vi "VIP_Post-Install Custom Action.vi"(10 "Variant":variant) -> (0 "error out":errorcluster)   [LabVIEW 2020]
uses:
  <vilib>/Utility/sysdir.llb/System Directory Type.ctl
  <userlib>/_OpenG.lib/file/file.llb/openg_file.lvlib
  <userlib>/_OpenG.lib/file/file.llb/Build Path - Traditional__ogtk.vi
  <userlib>/_OpenG.lib/lvzip/fileutil.llb/subVIs/FILE Rename (Path)__ogtk.vi
  <userlib>/_OpenG.lib/file/file.llb/File Exists - Scalar__ogtk.vi
panel:
  # "POST INSTALL"
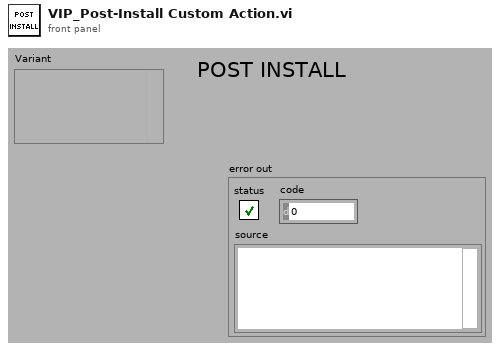
[diagram p1: front panel]
types:
  T1 = enum16{"open", "replace", "create", "open or create", "replace or create", "replace or create with confirmation"}
  T2 = typedef "System Directory Type.ctl" = i32
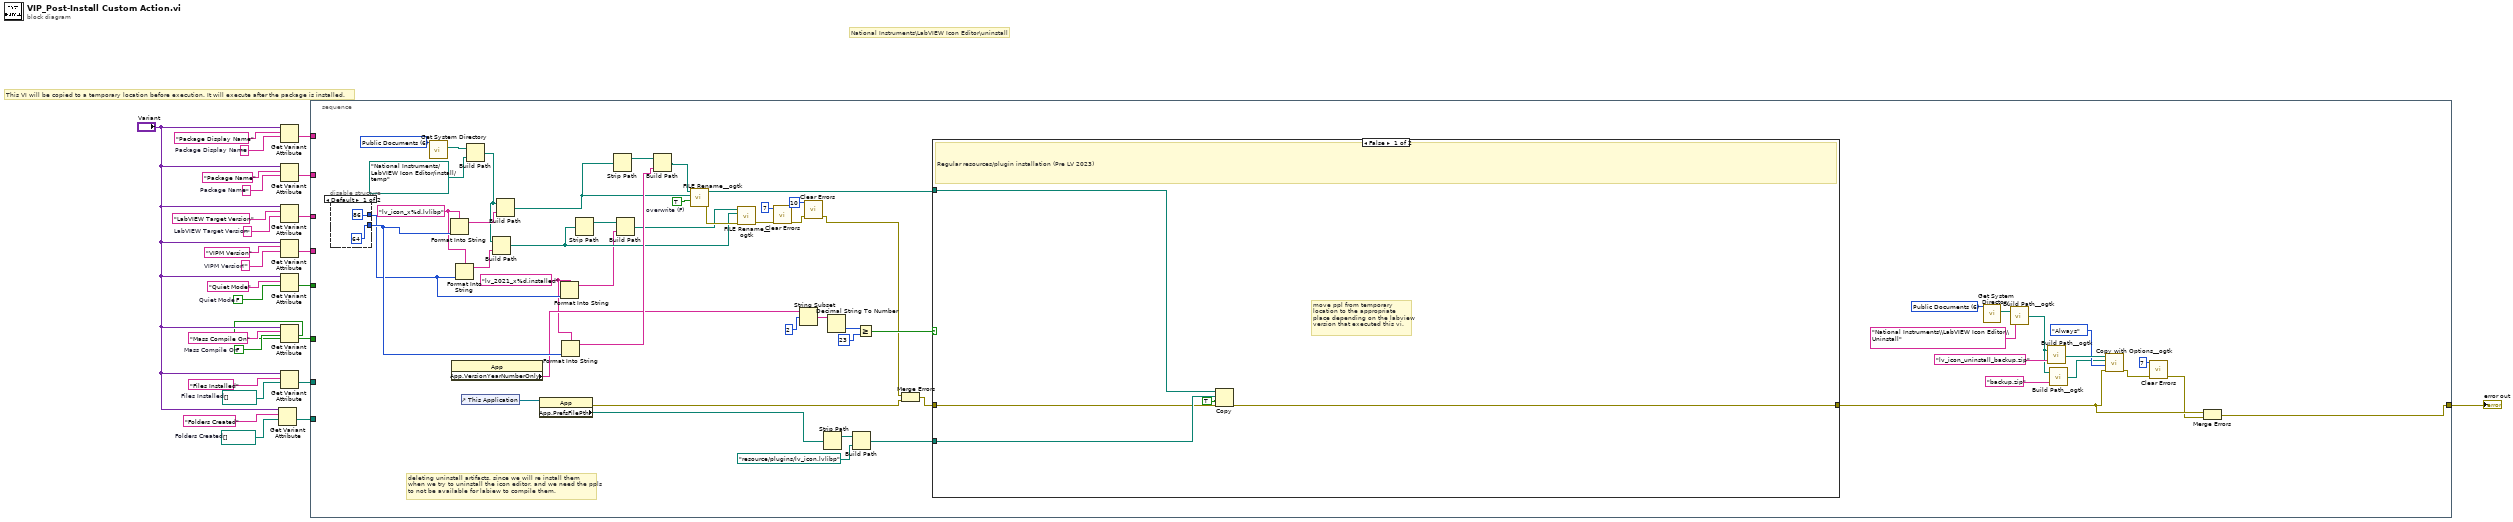
[diagram p0: block diagram]
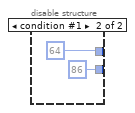
[diagram p2: hidden frame]
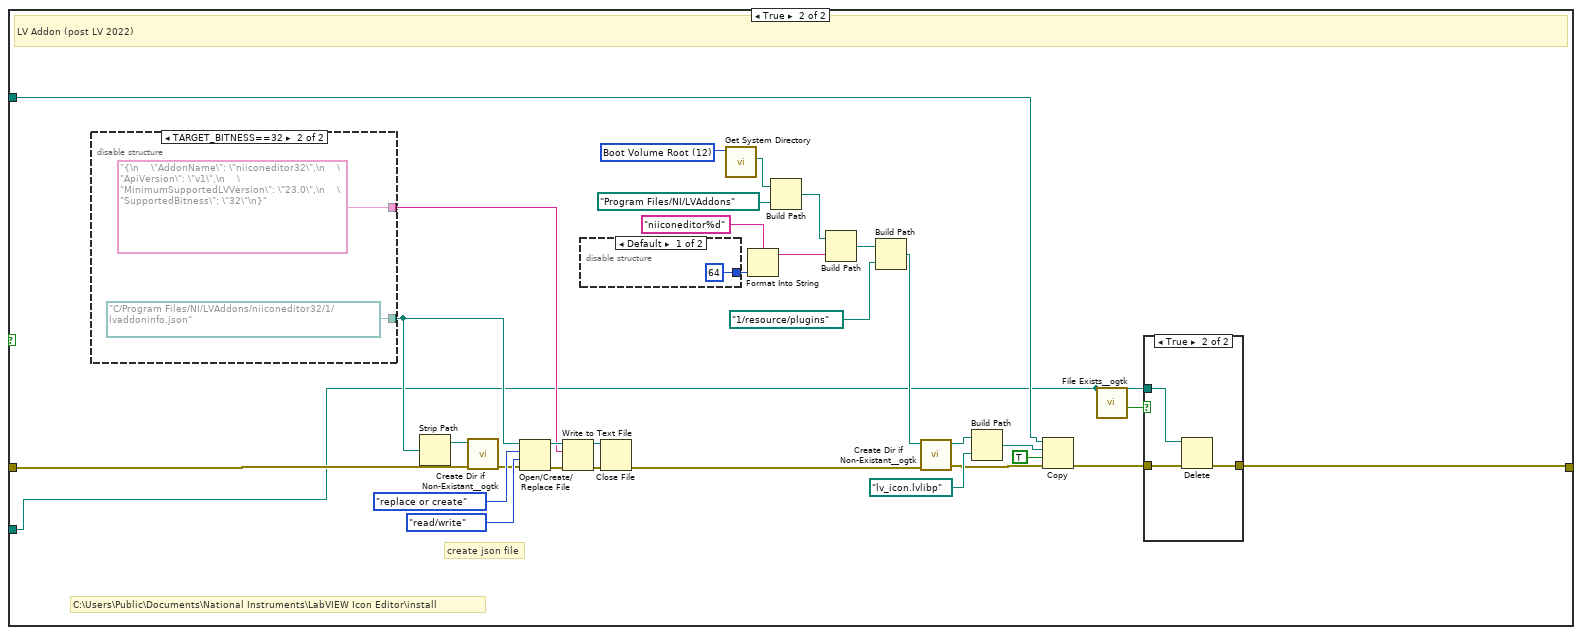
[diagram p3: hidden frame]
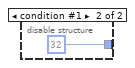
[diagram p5: hidden frame]
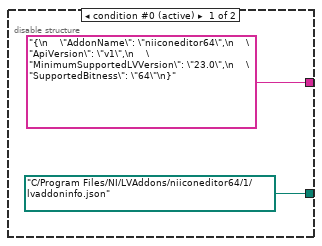
[diagram p6: hidden frame]
diagram:
  w10 = path[] []  # Folders Created
  w11 = path[] []  # Files Installed
  w15 = FALSE  # Mass Compile On
  w16 = ""  # Package Display Name
  w17 = FALSE  # Quiet Mode
  w20 = ""  # VIPM Version
  w22 = ""  # LabVIEW Target Version
  w24 = ""  # Package Name
  # "National Instruments\\LabVIEW Icon Editor\\uninstall"
  # "This VI will be copied to a temporary location before execution. It will execute after the package is installed."
  n1 = Get Variant Attribute(Variant="Variant", name="Folders Created", default value (empty Variant)=w10) -> (value=w2:path[])  [unwired: 1 in, 3 out]
  n2 = Get Variant Attribute(Variant="Variant", name="Package Display Name", default value (empty Variant)=w16) -> (value=w9:string)  [unwired: 1 in, 3 out]
  n3 = Get Variant Attribute(Variant="Variant", name="Package Name", default value (empty Variant)=w24) -> (value=w8:string)  [unwired: 1 in, 3 out]
  n4 = Get Variant Attribute(Variant="Variant", name="LabVIEW Target Version", default value (empty Variant)=w22) -> (value=w7:string)  [unwired: 1 in, 3 out]
  n5 = Get Variant Attribute(Variant="Variant", name="VIPM Version", default value (empty Variant)=w20) -> (value=w6:string)  [unwired: 1 in, 3 out]
  n6 = Get Variant Attribute(Variant="Variant", name="Quiet Mode", default value (empty Variant)=w17) -> (value=w5:bool)  [unwired: 1 in, 3 out]
  n7 = Get Variant Attribute(Variant="Variant", name="Mass Compile On", default value (empty Variant)=w15) -> (value=w4:bool)  [unwired: 1 in, 3 out]
  n8 = Get Variant Attribute(Variant="Variant", name="Files Installed", default value (empty Variant)=w11) -> (value=w3:path[])  [unwired: 1 in, 3 out]
  n9 = stacked-sequence {
    tunnel: [w28] -> w1
    tunnel: w9 -> [_]
    tunnel: w8 -> [_]
    tunnel: w7 -> [_]
    tunnel: w6 -> [_]
    tunnel: w5 -> [_]
    tunnel: w4 -> [_]
    tunnel: w3 -> [_]
    tunnel: w2 -> [_]
    frame #0 {
      w37 = "lv_2021_x%d.installed" ("format string")
      w57 = TRUE  # overwrite (F)
      w36 = "lv_icon_x%d.lvlibp" ("format string")
      w67 = T2 6 items=["User Home"=0, "User Desktop"=1, "User Documents"=2, "User Application Data"=3, "User Preferences"=4, "User Temporary"=5, "Public Documents"=6, "Public Application Data"=7, "Public Preferences"=8, "Public Cache"=13, "System Core Libraries"=9, "System Installed Libraries"=10, "Application Files"=11, "Boot Volume Root"=12] ("system directory type")
      w79 = T2 6 items=["User Home"=0, "User Desktop"=1, "User Documents"=2, "User Application Data"=3, "User Preferences"=4, "User Temporary"=5, "Public Documents"=6, "Public Application Data"=7, "Public Preferences"=8, "Public Cache"=13, "System Core Libraries"=9, "System Installed Libraries"=10, "Application Files"=11, "Boot Volume Root"=12] ("system directory type")
      # "deleting uninstall artifacts, since we will re install them\nwhen we try to uninstall the icon editor, and we need the ppls\nto not be available for labiew to compile them."
      n10 = disable-structure shown="Default" {
        disable-tunnel: [64 ("code") 86 ("code")] -> w56
        disable-tunnel: [86 ("code") 64 ("code")] -> w42
        frame condition #0 (active) {
        }
        frame condition #1 {
        }
      }
      n11 = call <vilib>:"Get System Directory.vi"("system directory type"=w79) -> ("system directory"=w55:path)  [unwired: 10 in]
      n12 = Format Into String(format string=w36, w56) -> (resulting string=w53:string)  [unwired: 2 in, 1 out]
      n13 = property class="App"() -> ("App.VersionYearNumberOnly"=w43:string)  [unwired: 2 in, 2 out]
      n14 = Format Into String(format string=w36, w42) -> (resulting string=w47:string)  [unwired: 2 in, 1 out]
      n15 = control-ref of="This Application"() -> (w78:refnum<vi>)
      n16 = Build Path(base path=w55, name or relative path=path "National Instruments/LabVIEW Icon Editor/install/temp" ("source path")) -> (appended path=w48:path)
      n17 = Build Path(base path=w48, name or relative path=w47) -> (appended path=w44:path)
      n18 = Build Path(base path=w48, name or relative path=w53) -> (appended path=w27:path)
      n19 = property class="App"(reference=w78) -> (error out=w58:errorcluster, "App.PrefsFilePth"=w62:path)  [unwired: 1 in, 1 out]
      n20 = Format Into String(format string=w37, w42) -> (resulting string=w41:string)  [unwired: 2 in, 1 out]
      n21 = Format Into String(format string=w37, w56) -> (resulting string=w50:string)  [unwired: 2 in, 1 out]
      n22 = Strip Path(path=w44) -> (stripped path=w45:path)  [unwired: 1 out]
      n23 = Strip Path(path=w27) -> (stripped path=w51:path)  [unwired: 1 out]
      n24 = Build Path(base path=w45, name or relative path=w41) -> (appended path=w40:path)
      n25 = Build Path(base path=w51, name or relative path=w50) -> (appended path=w49:path)
      n26 = call-poly <userlib>:"FILE Rename__ogtk.vi"("overwrite (F)"=w57, "source path"=w27, "target path"=w49) -> ("error out"=w46:errorcluster, "dup target path"=w52:path)  [unwired: 7 in]
      n27 = call-poly <userlib>:"FILE Rename__ogtk.vi"("error in (no error)"=w46, "source path"=w44, "target path"=w40) -> ("error out"=w39:errorcluster)  [unwired: 7 in, 1 out]
      n28 = call <vilib>:"Clear Errors.vi"("error in (no error)"=w39, "specific error code to clear (0: all)"=7) -> ("error out"=w35:errorcluster)  [unwired: 4 in, 1 out]
      n29 = String Subset(string=w43, offset (0)=2) -> (substring=w74:string)  [unwired: 1 in]
      n30 = call <vilib>:"Clear Errors.vi"("error in (no error)"=w35, "specific error code to clear (0: all)"=10) -> ("error out"=w34:errorcluster)  [unwired: 4 in, 1 out]
      n31 = Strip Path(path=w62) -> (stripped path=w64:path)  [unwired: 1 out]
      n32 = Decimal String To Number(string=w74) -> (number=w75:i32)  [unwired: 2 in, 1 out]
      n33 = Build Path(base path=w64, name or relative path=path "resource/plugins/lv_icon.lvlibp") -> (appended path=w61:path)
      n34 = Greater Or Equal?(x=w75, y=23) -> (x >= y?=w76:bool)
      n35 = Merge Errors(w34, w58) -> (w60:errorcluster)
      n36 = case shown="False" w76 {
        tunnel: w52 -> [w84 w92]
        tunnel: w60 -> [w85 w97]
        tunnel: w61 -> [w88 w90]
        tunnel: [w86 w96] -> w30
        frame False {
          # "move ppl from temporary\nlocation to the appropriate\nplace depending on the labview\nversion that executed this vi."
          # "Regular resources/plugin installation (Pre LV 2023)"
          n37 = Copy(8:w85, 9:TRUE ("overwrite (F)"), 10:w88, 11:w84) -> (0:w86:errorcluster)  [unwired: 1 in, 2 out]
        }
        frame True {
          w106 = T2 12 items=["User Home"=0, "User Desktop"=1, "User Documents"=2, "User Application Data"=3, "User Preferences"=4, "User Temporary"=5, "Public Documents"=6, "Public Application Data"=7, "Public Preferences"=8, "Public Cache"=13, "System Core Libraries"=9, "System Installed Libraries"=10, "Application Files"=11, "Boot Volume Root"=12] ("system directory type")
          # "C:\\Users\\Public\\Documents\\National Instruments\\LabVIEW Icon Editor\\install"
          # "create json file"
          # "LV Addon (post LV 2022)"
          n38 = disable-structure shown="TARGET_BITNESS==32" {
            disable-tunnel: [path "C:/Program Files/NI/LVAddons/niiconeditor64/1/lvaddoninfo.json" ("Destination[i] Paths (Absolute)") path "C:/Program Files/NI/LVAddons/niiconeditor32/1/lvaddoninfo.json" ("Destination[i] Paths (Absolute)")] -> w103
            disable-tunnel: ["{\n    \"AddonName\": \"niiconeditor64\",\n    \"ApiVersion\": \"v1\",\n    \"MinimumSupportedLVVersion\": \"23.0\",\n    \"SupportedBitness\": \"64\"\n}" ("Tag Name") "{\n    \"AddonName\": \"niiconeditor32\",\n    \"ApiVersion\": \"v1\",\n    \"MinimumSupportedLVVersion\": \"23.0\",\n    \"SupportedBitness\": \"32\"\n}" ("Tag Name")] -> w114
            frame condition #0 (active) {
            }
            frame condition #1 {
            }
          }
          n39 = Strip Path(path=w103) -> (stripped path=w102:path)  [unwired: 1 out]
          n40 = call <userlib>:"Create Dir if Non-Existant__ogtk.vi"("error in (no error)"=w97, "Directory Path"=w102) -> ("error out"=w101:errorcluster)  [unwired: 7 in, 2 out]
          n41 = Open/Create/Replace File(file path (use dialog)=w103, error in=w101, operation (0:open)=T1."replace or create", access (0:read/write)=enum16{"read/write", "read-only", "write-only"}."read/write") -> (refnum out=w118:refnum<file>, error out=w119:errorcluster)  [unwired: 2 in, 1 out]
          n42 = Write to Text File(file (use dialog)=w118, text=w114, error in=w119) -> (refnum out=w117:refnum<file>, error out=w120:errorcluster)  [unwired: 1 in, 1 out]
          n43 = disable-structure shown="Default" {
            disable-tunnel: [64 ("code") 32 ("code")] -> w109
            frame condition #0 (active) {
            }
            frame condition #1 {
            }
          }
          n44 = Close File(refnum=w117, error in=w120) -> (error out=w98:errorcluster)  [unwired: 1 out]
          n45 = call <vilib>:"Get System Directory.vi"("system directory type"=w106) -> ("system directory"=w110:path)  [unwired: 10 in]
          n46 = Format Into String(format string="niiconeditor%d", w109) -> (resulting string=w112:string)  [unwired: 2 in, 1 out]
          n47 = Build Path(base path=w110, name or relative path=path "Program Files/NI/LVAddons") -> (appended path=w111:path)
          n48 = Build Path(base path=w111, name or relative path=w112) -> (appended path=w113:path)
          n49 = Build Path(base path=w113, name or relative path=path "1/resource/plugins") -> (appended path=w100:path)
          n50 = call <userlib>:"Create Dir if Non-Existant__ogtk.vi"("error in (no error)"=w98, "Directory Path"=w100) -> ("error out"=w94:errorcluster, "dup Directory Path"=w99:path)  [unwired: 7 in, 1 out]
          n51 = Build Path(base path=w99, name or relative path=path "lv_icon.lvlibp" ("source path")) -> (appended path=w91:path)
          n52 = Copy(8:w94, 9:TRUE ("overwrite (F)"), 10:w91, 11:w92) -> (0:w89:errorcluster)  [unwired: 1 in, 2 out]
          n53 = call-poly <userlib>:"File Exists__ogtk.vi"("file path"=w90) -> ("exists"=w95:bool)  [unwired: 6 in, 1 out]
          n54 = case shown="True" w95 {
            tunnel: w89 -> [w121 w124]
            tunnel: w90 -> [_ w123]
            tunnel: [w121 w122] -> w96
            frame False {
            }
            frame True {
              n55 = Delete(path (use dialog)=w123, error in=w124) -> (error out=w122:errorcluster)  [unwired: 3 in, 2 out]
            }
          }
        }
      }
      n56 = call <vilib>:"Get System Directory.vi"("system directory type"=w67) -> ("system directory"=w71:path)  [unwired: 10 in]
      n57 = call-poly <userlib>:"Build Path__ogtk.vi"("name or relative path"="National Instruments\\LabVIEW Icon Editor\\Uninstall", "base path"=w71) -> ("appended path"=w59:path)
      n58 = call-poly <userlib>:"Build Path__ogtk.vi"("name or relative path"="lv_icon_uninstall_backup.zip", "base path"=w59) -> ("appended path"=w72:path)
      n59 = call-poly <userlib>:"Build Path__ogtk.vi"("name or relative path"="backup.zip", "base path"=w59) -> ("appended path"=w65:path)
      n60 = call <userlib>:"Copy with Options__ogtk.vi"("error in (no error)"=w30, "Replace Mode (Never)"=enum16{"Never", "Always", "If Newer"}."Always", "target path"=w65, "source path"=w72) -> ("error out"=w32:errorcluster)  [unwired: 6 in, 1 out]
      n61 = call <vilib>:"Clear Errors.vi"("error in (no error)"=w32, "specific error code to clear (0: all)"=7) -> ("error out"=w29:errorcluster)  [unwired: 4 in, 1 out]
      n62 = Merge Errors(w30, w29) -> (w28:errorcluster)
    }
  }
  "error out" <- w1
